vi "Handle Error.vi"(7 "Stop on Unhandled Error (T)":bool=TRUE, 8 "error in":errorcluster, 11 "Instrument.Oxford1820 UI":refnum<class "Instrument UI.Oxford1820.lvclass">) -> (0 "handling error":errorcluster, 2 "Unhandled error":errorcluster, 3 "Instrument.Oxford1820 UI out":refnum<class "Instrument UI.Oxford1820.lvclass">)   [LabVIEW 2016, in "Instrument UI.Oxford1820.lvclass"]
doc: "JKI State Machine Objects (SMO) 1.0.0.11\nJKI - JKI\nCopyright (c) 2016, JKIJKI State Machine Objects (SMO) 1.3.0.56\nJKI - JKI\nCopyright (c) 2017, JKI"
uses:
  Instrument UI.Oxford1820.lvclass
  <userlib>/LevyLab/Levylab Instruments/SMOs/Instrument UI/Instrument UI.lvclass
  <userlib>/LevyLab/Levylab Instruments/SMOs/Logger.Error/Logger.Error.lvclass
panel:
  # "For instructions on how to use the JKI State Machine Objects, examples and video tutorials, visit:\nhttp://jki.net/state-machine-objects/\n\nJKI State Machine Objects™\nhttp://jki.net/state-machine-objects/\nCopyright (C) 2005-2015, JKI <info@jki.net>\nALL RIGHTS RESERVED"
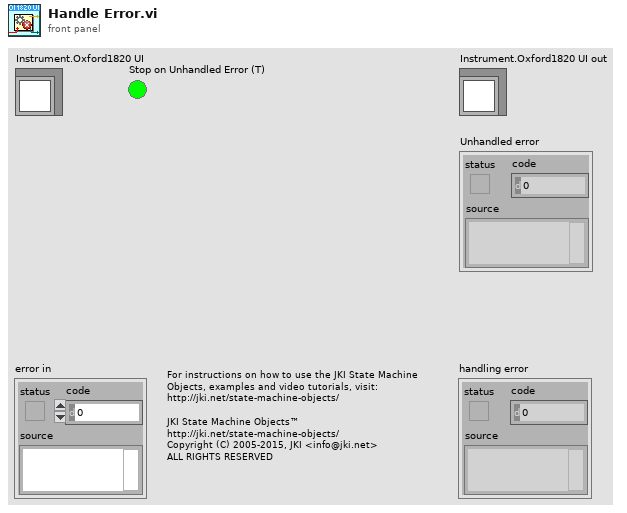
[diagram p1: front panel]
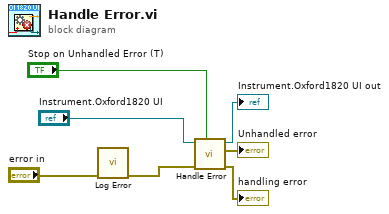
[diagram p0: block diagram]
diagram:
  n1 = call <userlib>:"Log Error.vi"("error in (no error)"="error in") -> ("error out"=w1:errorcluster)  [unwired: 9 in, 1 out]
  n2 = call-parent "Handle Error.vi"("Stop on Unhandled Error (T)"="Stop on Unhandled Error (T)", "error in"=w1, "Instrument UI"="Instrument.Oxford1820 UI") -> ("handling error"=→"handling error":errorcluster, "Unhandled error"=→"Unhandled error":errorcluster, "Instrument UI out"=→"Instrument.Oxford1820 UI out":refnum<class "Instrument UI.Oxford1820.lvclass">)  [unwired: 6 in]
